vi "CleanJoystickAnalogValues.vi"(8 "Cube Outputs?":bool, 9 "Lower threshold":dbl=-0.1, 10 "Upper threshold":dbl=0.1, 11 "Numbers":dbl[](array[numeric])) -> (3 "Corrected numbers":dbl[](array[numeric]))   [LabVIEW 2014]
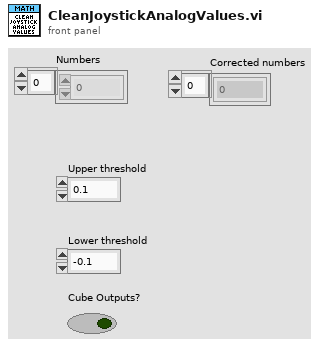
[diagram p1: front panel]
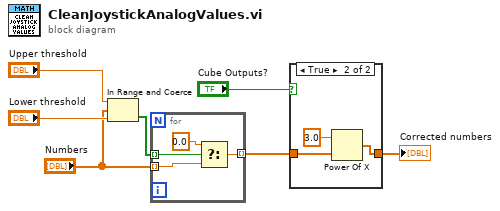
[diagram p0: block diagram]
diagram:
  n1 = In Range and Coerce(upper limit="Upper threshold", x="Numbers", lower limit="Lower threshold") -> (In Range?=w4:bool[])  [unwired: 1 out]
  n2 = for {
    tunnel: w4 -> [w11] mode=indexing
    tunnel: "Numbers" -> [w10] mode=indexing
    tunnel: [w8] -> w2 mode=indexing
    n3 = Select(t=0.0, s=w11, f=w10) -> (s? t:f=w8:dbl)
  }
  n4 = case shown="True" "Cube Outputs?" {
    tunnel: w2 -> [w12 w15]
    tunnel: [w12 w13] -> w1
    frame False {
    }
    frame True {
      n5 = Power Of X(1:w15, 2:3.0) -> (0:w13:dbl[])
    }
  }
  "Corrected numbers" <- w1
